vi "HH_ToImage_2.vi"(0 "Data In":u32[](array[numeric]), 1 "Reset":bool, 2 "Image Data In":u16[][](array[numeric]), 5 "Data Count":i32, 7 "Trigger Times":u64[](array[numeric]), 9 "Trigger":dbl[](array[numeric])) -> (3 "Image Data Out":u16[][](array[numeric]), 6 "Total Photon Count":u64[](array[numeric]), 13 "Total Oveflow Count":u64, 14 "Num Records Total":i64)   [LabVIEW 2011]
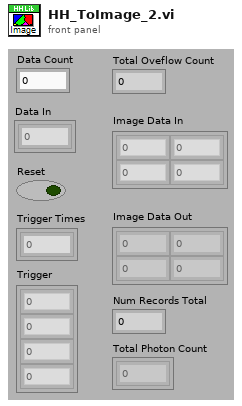
[diagram p1: front panel]
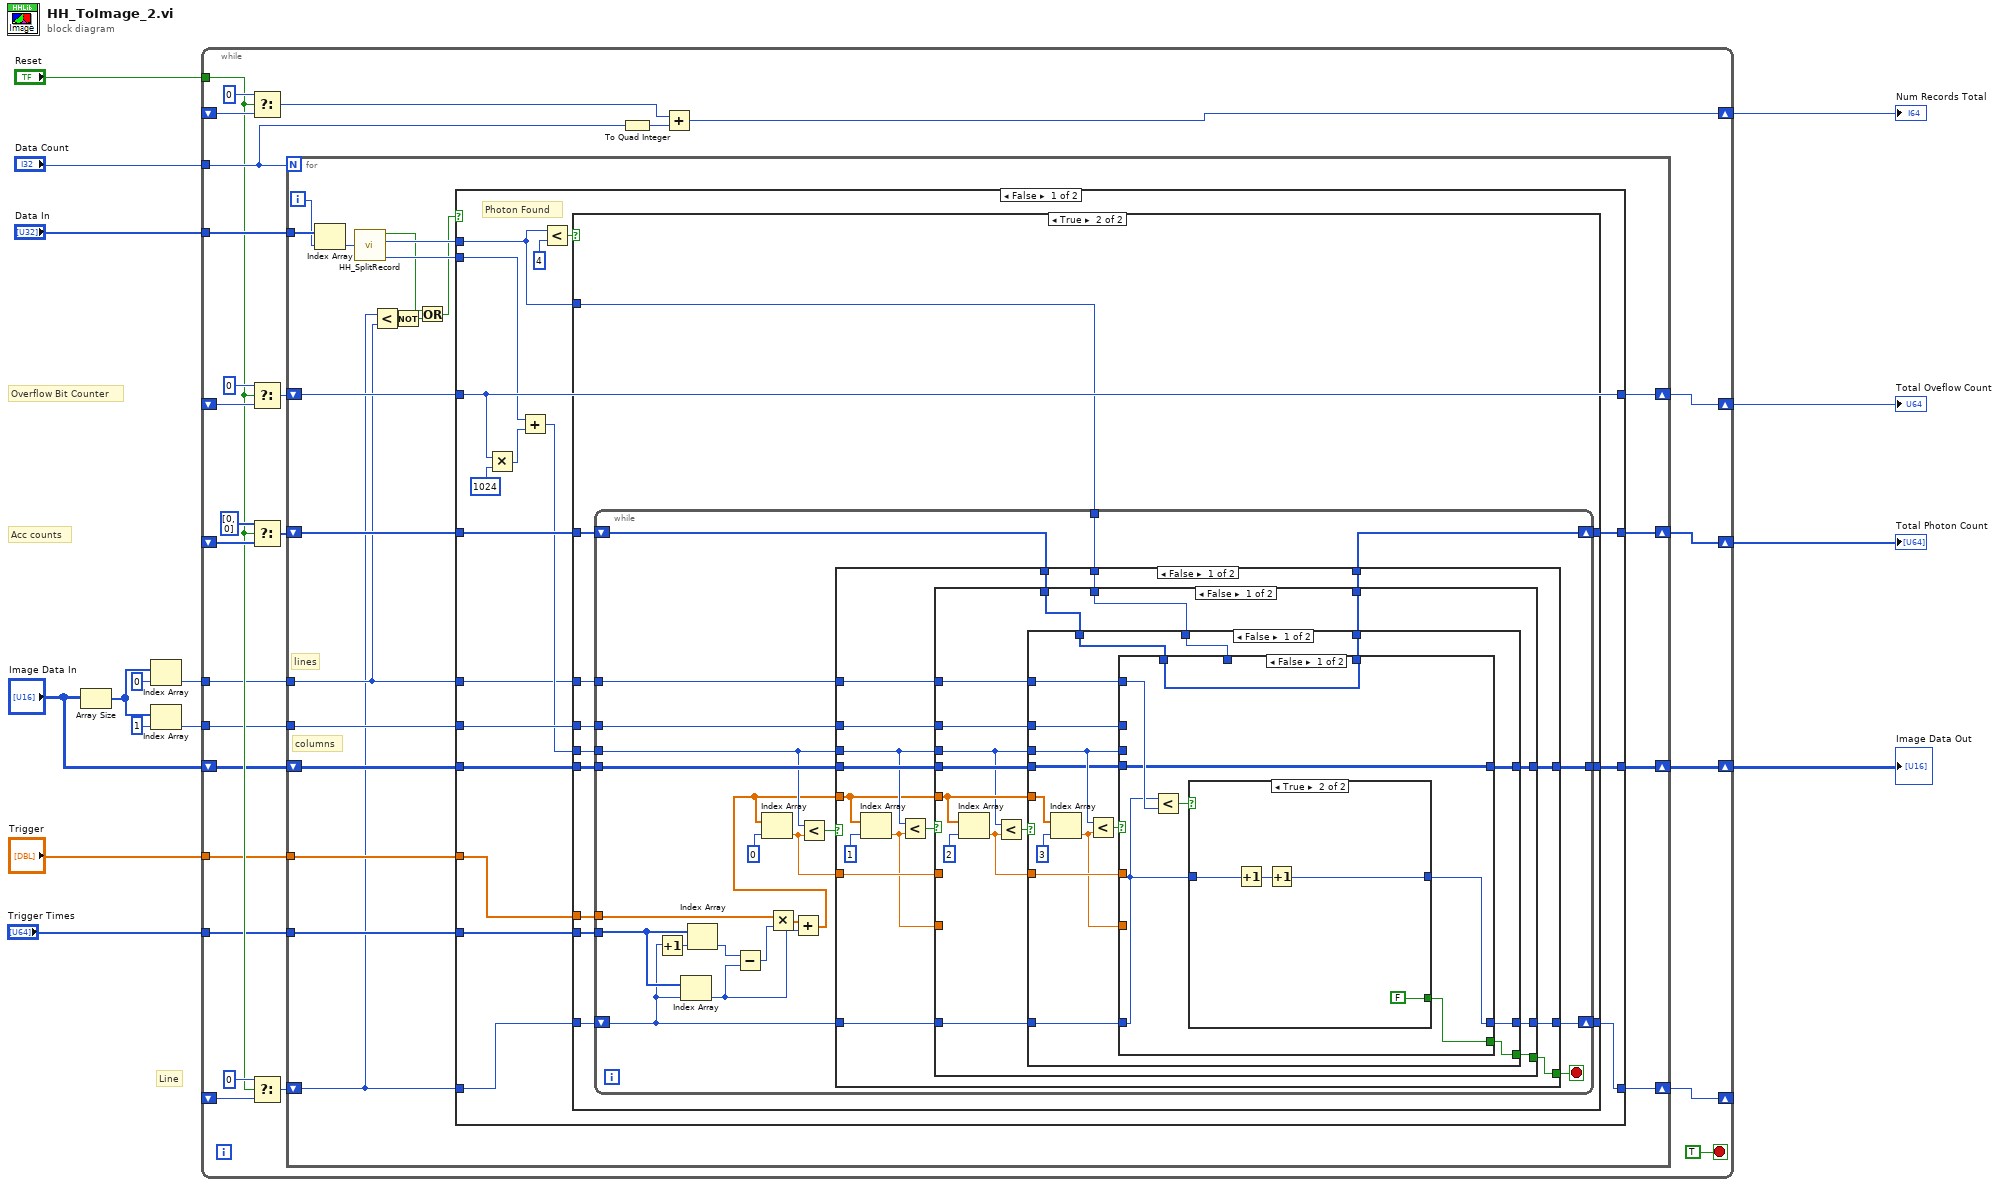
[diagram p0: block diagram]
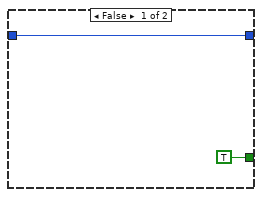
[diagram p3: hidden frame]
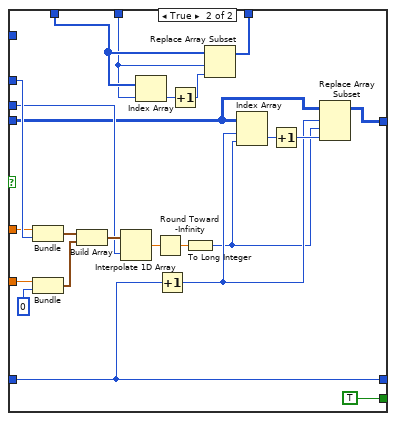
[diagram p4: hidden frame]
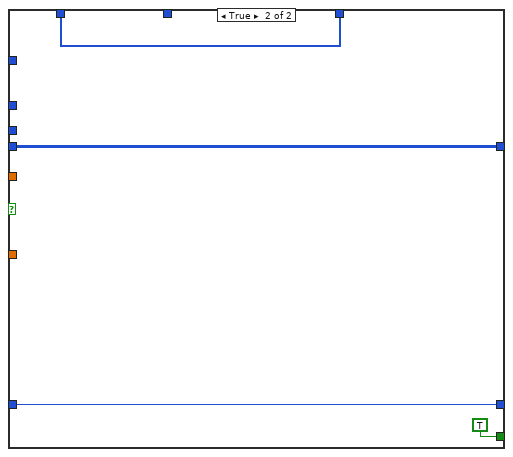
[diagram p5: hidden frame]
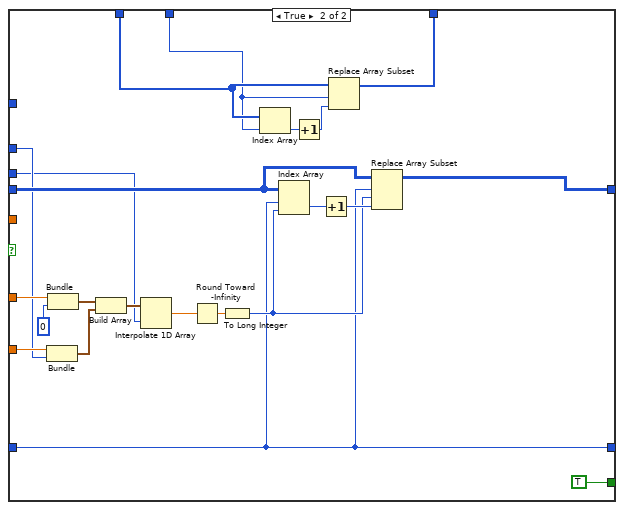
[diagram p6: hidden frame]
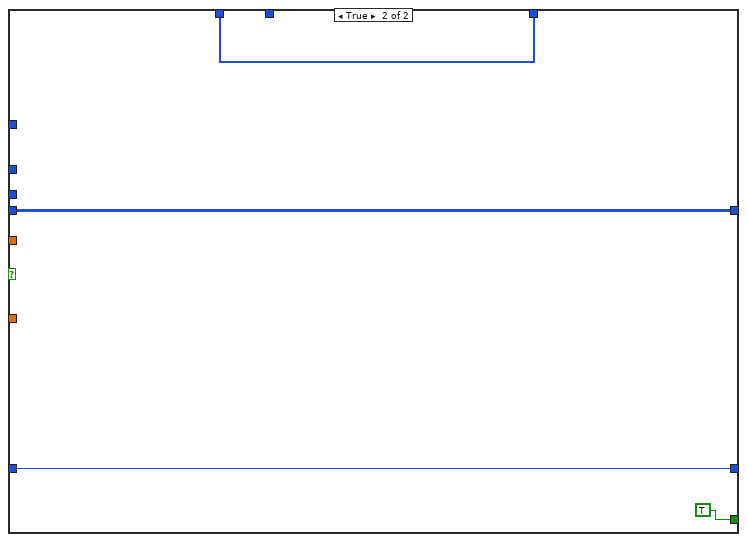
[diagram p7: hidden frame]
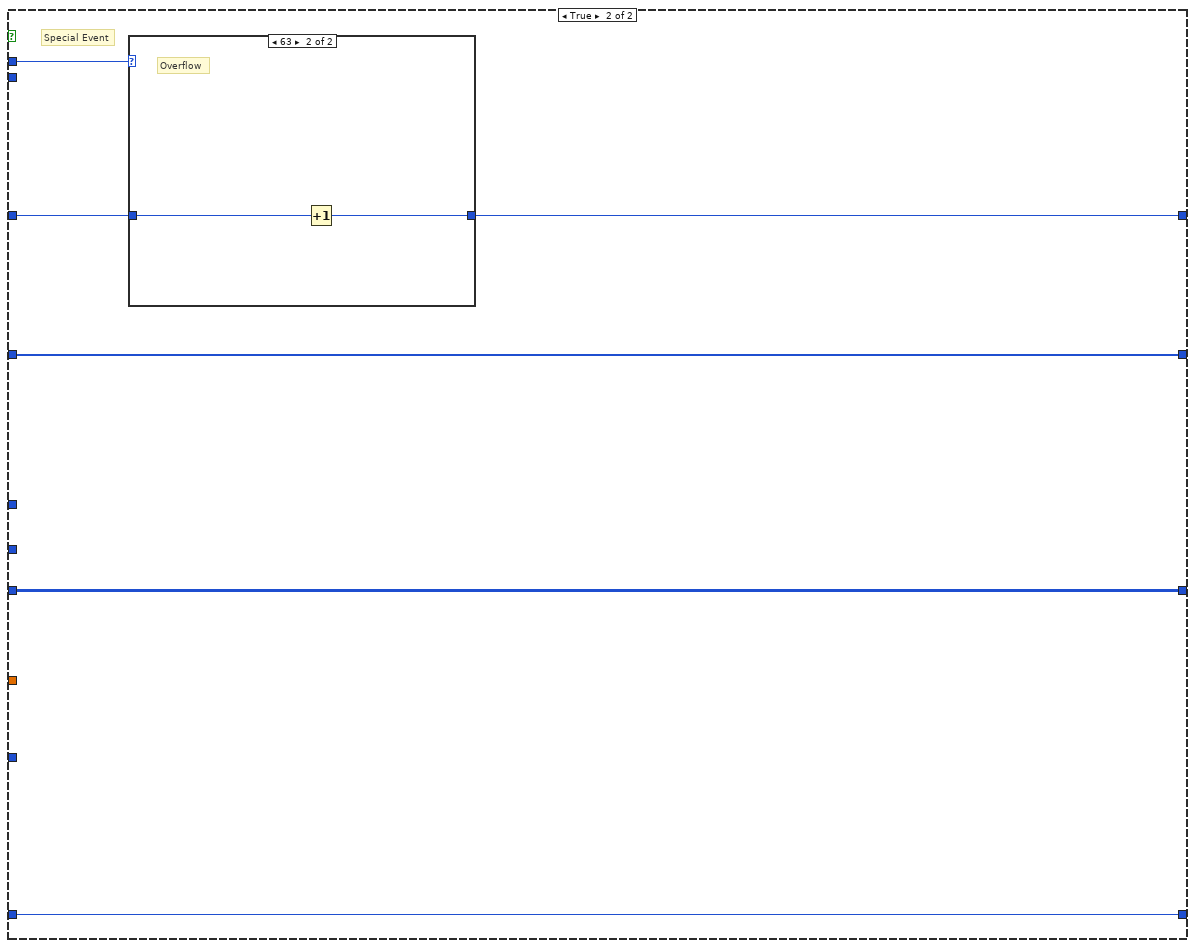
[diagram p8: hidden frame]
diagram:
  # "Line"
  # "Acc counts"
  # "Overflow Bit Counter"
  n1 = Array Size(array="Image Data In") -> (size(s)=w8:i32[])
  n2 = Index Array(array=w8, index=0) -> (element=w3:i32)
  n3 = Index Array(array=w8, index=1) -> (element=w4:i32)
  n4 = while {
    tunnel: "Data In" -> [w42]
    tunnel: "Reset" -> [w22]
    shift-right: [w38] -> w11
    shift-left: _ -> [w37]
    shift-right: [w34] -> _
    shift-left: _ -> [w21]
    tunnel: "Data Count" -> [w25]
    shift-right: [w30] -> w12
    shift-left: _ -> [w32]
    shift-right: [w27] -> w10
    shift-left: _ -> [w26]
    shift-right: [w23] -> w2
    shift-left: "Image Data In" -> [w20]
    tunnel: "Trigger Times" -> [w18]
    tunnel: w4 -> [w19]
    tunnel: w3 -> [w16]
    tunnel: "Trigger" -> [w17]
    stop <- TRUE stop-if-true
    n5 = Select(t=i64 0 ("Data Count 2"), s=w22, f=w32) -> (s? t:f=w31:i64)
    n6 = Select(t=u64 0, s=w22, f=w37) -> (s? t:f=w39:u64)
    n7 = Select(t=u64[] [0, 0] ("initialized array"), s=w22, f=w26) -> (s? t:f=w28:u64[])
    n8 = Select(t=0, s=w22, f=w21) -> (s? t:f=w35:i32)
    n9 = for {
      N: w25 -> [_]
      tunnel: w42 -> [w61]
      shift-right: [w62] -> w38
      shift-left: w39 -> [w63]
      shift-right: [w53] -> w34
      shift-left: w35 -> [w47]
      shift-right: [w58] -> w27
      shift-left: w28 -> [w59]
      shift-right: [w54] -> w23
      shift-left: w20 -> [w55]
      tunnel: w19 -> [w49]
      tunnel: w18 -> [w50]
      tunnel: w17 -> [w51]
      tunnel: w16 -> [w48]
      i -> [w60]
      # "lines"
      # "columns"
      n10 = Index Array(array=w61, index=w60) -> (element=w57:u32)
      n11 = call "HH_SplitRecord.vi"("Record in"=w57) -> ("Special"=w45:bool, "channel"=w56:i32, "nsync"=w52:u16)  [unwired: 1 out]
      n12 = Less?(x=w47, y=w48) -> (x < y?=w46:bool)
      n13 = Not(x=w46) -> (.not. x?=w43:bool)
      n14 = Or(x=w45, y=w43) -> (x .or. y?=w44:bool)
      n15 = case shown="False" w44 {
        tunnel: w56 -> [w73 w234]
        tunnel: w63 -> [w76 w233]
        tunnel: [w76 w232] -> w62
        tunnel: w52 -> [w71 _]
        tunnel: w59 -> [w79 w235]
        tunnel: [w78 w235] -> w58
        tunnel: w47 -> [w65 w237]
        tunnel: w55 -> [w77 w236]
        tunnel: [w72 w236] -> w54
        tunnel: [w69 w237] -> w53
        tunnel: w51 -> [w68 _]
        tunnel: w50 -> [w67 _]
        tunnel: w49 -> [w70 _]
        tunnel: w48 -> [w64 _]
        frame False {
          # "Photon Found"
          n16 = Multiply(x=w76, y=1024) -> (x*y=w74:u64)
          n17 = Add(x=w71, y=w74) -> (x+y=w66:u64)
          n18 = Less?(x=w73, y=4) -> (x < y?=w81:bool)
          n19 = case shown="True" w81 {
            tunnel: w73 -> [_ w85]
            tunnel: w79 -> [w83 w87]
            tunnel: [w83 w86] -> w78
            tunnel: w77 -> [w84 w96]
            tunnel: [w84 w95] -> w72
            tunnel: w66 -> [_ w94]
            tunnel: w65 -> [w82 w93]
            tunnel: w70 -> [_ w92]
            tunnel: [w82 w91] -> w69
            tunnel: w64 -> [_ w90]
            tunnel: w68 -> [_ w89]
            tunnel: w67 -> [_ w88]
            frame False {
            }
            frame True {
              n20 = while {
                tunnel: w96 -> [w118]
                tunnel: [w117] -> w95
                tunnel: w94 -> [w114]
                tunnel: w92 -> [w113]
                shift-right: [w111] -> w91
                shift-left: w93 -> [w97]
                tunnel: w90 -> [w109]
                tunnel: w89 -> [w102]
                tunnel: w88 -> [w101]
                tunnel: w85 -> [w98]
                shift-right: [w99] -> w86
                shift-left: w87 -> [w100]
                stop <- w115 stop-if-true
                n21 = Increment(x=w97) -> (x+1=w108:i32)
                n22 = Index Array(array=w101, index=w97) -> (element=w105:u64)
                n23 = Index Array(array=w101, index=w108) -> (element=w107:u64)
                n24 = Subtract(x=w107, y=w105) -> (x-y=w106:u64)
                n25 = Multiply(x=w102, y=w106) -> (x*y=w104:dbl[])
                n26 = Add(x=w104, y=w105) -> (x+y=w103:dbl[])
                n27 = Index Array(array=w103, index=0) -> (element=w112:dbl)
                n28 = Less?(x=w114, y=w112) -> (x < y?=w116:bool)
                n29 = case shown="False" w116 {
                  tunnel: w118 -> [w132 w231]
                  tunnel: [w131 w231] -> w117
                  tunnel: w103 -> [w124 _]
                  tunnel: [w123 TRUE] -> w115
                  tunnel: w114 -> [w126 _]
                  tunnel: w97 -> [w130 w229]
                  tunnel: w113 -> [w129 _]
                  tunnel: w112 -> [w128 _]
                  tunnel: [w125 w229] -> w111
                  tunnel: w109 -> [w122 _]
                  tunnel: w100 -> [w121 w228]
                  tunnel: [w120 w228] -> w99
                  tunnel: w98 -> [w119 _]
                  frame False {
                    n30 = Index Array(array=w124, index=1) -> (element=w127:dbl)
                    n31 = Less?(x=w126, y=w127) -> (x < y?=w133:bool)
                    n32 = case shown="False" w133 {
                      tunnel: w132 -> [w144 w225]
                      tunnel: [w143 w224] -> w131
                      tunnel: w130 -> [w147 w212]
                      tunnel: w129 -> [w139 w218]
                      tunnel: w128 -> [_ w221]
                      tunnel: w127 -> [_ w220]
                      tunnel: w126 -> [w141 w213]
                      tunnel: [w146 w212] -> w125
                      tunnel: w124 -> [w142 _]
                      tunnel: [w145 TRUE] -> w123
                      tunnel: w122 -> [w138 _]
                      tunnel: w121 -> [w136 w208]
                      tunnel: [w137 w207] -> w120
                      tunnel: w119 -> [w135 w206]
                      frame False {
                        n33 = Index Array(array=w142, index=2) -> (element=w140:dbl)
                        n34 = Less?(x=w141, y=w140) -> (x < y?=w148:bool)
                        n35 = case shown="False" w148 {
                          tunnel: w147 -> [w158 w205]
                          tunnel: [w157 w205] -> w146
                          tunnel: [w154 TRUE] -> w145
                          tunnel: w144 -> [w156 w203]
                          tunnel: [w155 w203] -> w143
                          tunnel: w142 -> [w164 _]
                          tunnel: w141 -> [w159 _]
                          tunnel: w140 -> [w162 _]
                          tunnel: w139 -> [w160 _]
                          tunnel: w138 -> [w153 _]
                          tunnel: [w150 w202] -> w137
                          tunnel: w136 -> [w152 w202]
                          tunnel: w135 -> [w151 _]
                          frame False {
                            n36 = Index Array(array=w164, index=3) -> (element=w161:dbl)
                            n37 = Less?(x=w159, y=w161) -> (x < y?=w163:bool)
                            n38 = case shown="False" w163 {
                              tunnel: w162 -> [_ w193]
                              tunnel: w161 -> [_ w195]
                              tunnel: w160 -> [_ w194]
                              tunnel: w159 -> [_ w192]
                              tunnel: w158 -> [w170 w189]
                              tunnel: [w169 w189] -> w157
                              tunnel: w156 -> [w167 w187]
                              tunnel: [w167 w186] -> w155
                              tunnel: [w168 TRUE] -> w154
                              tunnel: w153 -> [w172 _]
                              tunnel: w152 -> [w166 w181]
                              tunnel: w151 -> [_ w180]
                              tunnel: [w166 w179] -> w150
                              frame False {
                                n39 = Less?(x=w170, y=w172) -> (x < y?=w171:bool)
                                n40 = case shown="True" w171 {
                                tunnel: w170 -> [w174 w177]
                                tunnel: [w174 w176] -> w169
                                tunnel: [TRUE FALSE] -> w168
                                frame False {
                                }
                                frame True {
                                n41 = Increment(x=w177) -> (x+1=w178:i32)
                                n42 = Increment(x=w178) -> (x+1=w176:i32)
                                }
                                }
                              }
                              frame True {
                                n43 = Bundle(w193, w194) -> (w201:cluster{dbl, i32})  [unwired: 1 in]
                                n44 = Bundle(w195, 0) -> (w200:cluster{dbl, i32})  [unwired: 1 in]
                                n45 = Build Array(w201, w200) -> (w199:cluster{dbl, i32}[])
                                n46 = Interpolate 1D Array(1:w192, 2:w199) -> (0:w198:dbl)
                                n47 = Index Array(array=w181, index=w180) -> (element=w183:u64)
                                n48 = Round Toward -Infinity(1:w198) -> (0:w197:dbl)
                                n49 = Increment(x=w189) -> (x+1=w188:i32)
                                n50 = Increment(x=w183) -> (x+1=w182:u64)
                                n51 = To Long Integer(number=w197) -> (32bit integer=w185:i32)
                                n52 = Replace Array Subset(array=w181, new element=w182, index=w180) -> (w179:u64[])
                                n53 = Index Array(array=w187, index (row)=w188, index (col)=w185) -> (element=w191:u16)
                                n54 = Increment(x=w191) -> (x+1=w190:u16)
                                n55 = Replace Array Subset(array=w187, new element=w190, index (row)=w188, index (col)=w185) -> (w186:u16[][])
                              }
                            }
                          }
                          frame True {
                          }
                        }
                      }
                      frame True {
                        n56 = Bundle(w220, w218) -> (w222:cluster{dbl, i32})  [unwired: 1 in]
                        n57 = Bundle(w221, 0) -> (w223:cluster{dbl, i32})  [unwired: 1 in]
                        n58 = Build Array(w223, w222) -> (w217:cluster{dbl, i32}[])
                        n59 = Interpolate 1D Array(1:w213, 2:w217) -> (0:w216:dbl)
                        n60 = Round Toward -Infinity(1:w216) -> (0:w215:dbl)
                        n61 = To Long Integer(number=w215) -> (32bit integer=w214:i32)
                        n62 = Index Array(array=w208, index=w206) -> (element=w210:u64)
                        n63 = Index Array(array=w225, index (row)=w212, index (col)=w214) -> (element=w227:u16)
                        n64 = Increment(x=w210) -> (x+1=w209:u64)
                        n65 = Increment(x=w227) -> (x+1=w226:u16)
                        n66 = Replace Array Subset(array=w208, new element=w209, index=w206) -> (w207:u64[])
                        n67 = Replace Array Subset(array=w225, new element=w226, index (row)=w212, index (col)=w214) -> (w224:u16[][])
                      }
                    }
                  }
                  frame True {
                  }
                }
              }
            }
          }
        }
        frame True {
          # "Special Event"
          n68 = case shown="63" w234 {
            tunnel: w233 -> [w238 w240]
            tunnel: [w238 w239] -> w232
            frame Default {
            }
            frame 63 {
              # "Overflow"
              n69 = Increment(x=w240) -> (x+1=w239:u64)
            }
          }
        }
      }
    }
    n70 = To Quad Integer(1:w25) -> (0:w24:i64)
    n71 = Add(x=w31, y=w24) -> (x+y=w30:i64)
  }
  "Num Records Total" <- w12
  "Total Oveflow Count" <- w11
  "Total Photon Count" <- w10
  "Image Data Out" <- w2
